vi "Multi_Read_Single.vi"(6 "Manual Range (1)":dbl=1.0, 7 "Auto Range (T: Enable)":bool=TRUE, 8 "error in":errorcluster, 9 "Absolute Resolution (1E-6)":dbl=1e-06, 10 "Measurement Function (10: Voltage DC)":i32(ring)=10 items=["Continuity", "Current AC", "Current DC", "Diode", "Frequency", "Resistance 4-wire", "Period", "Resistance 2-wire", "Temperature", "Voltage AC", "Voltage DC", "Voltage DC Ratio"], 11 "VISA resource name":refnum<visa-resource-name>) -> (0 "error out":errorcluster, 2 "Measurement":dbl)   [LabVIEW 2015]
doc: "This example shows how to configure a measurement and take a reading."
uses:
  <instrlib>/Agilent 3446X Series/Public/Data/Read (Single Point).vi
  <instrlib>/Agilent 3446X Series/Agilent 3446X Series.lvlib
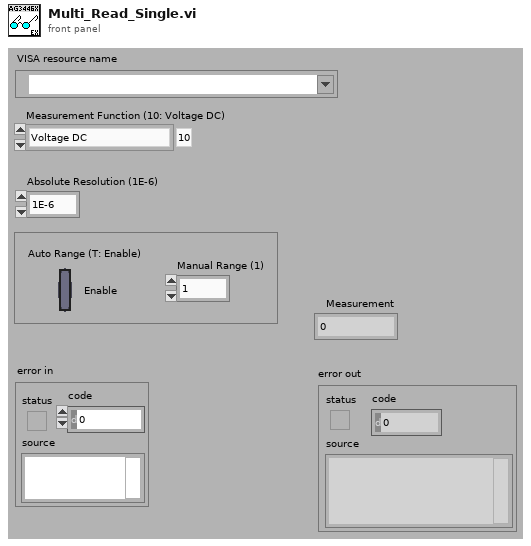
[diagram p1: front panel]
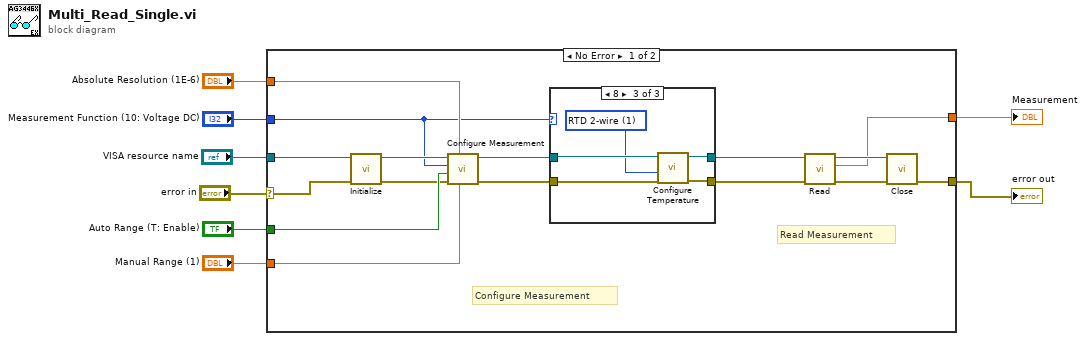
[diagram p0: block diagram]
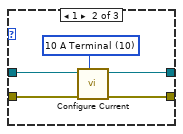
[diagram p3: hidden frame]
diagram:
  n1 = case shown="No Error" "error in" {
    selector: "error in" -> [w16 w37]
    tunnel: [w22 _] -> w8
    tunnel: "Measurement Function (10: Voltage DC)" -> [w9 _]
    tunnel: "Absolute Resolution (1E-6)" -> [w21 _]
    tunnel: "Auto Range (T: Enable)" -> [w20 _]
    tunnel: "Manual Range (1)" -> [w19 _]
    tunnel: "VISA resource name" -> [w18 _]
    tunnel: [w17 w37] -> w2
    frame No Error {
      # "Read Measurement"
      # "Configure Measurement"
      n2 = call <instrlib>:"Initialize.vi"("error in (no error)"=w16, "VISA resource name"=w18) -> ("error out"=w10:errorcluster, "VISA resource name out"=w11:refnum<visa-resource-name>)  [unwired: 3 in, 5 out]
      n3 = call <instrlib>:"Configure Measurement.vi"("Manual Range (1)"=w19, "Absolute Resolution (1E-6)"=w21, "error in (no error)"=w10, "Auto Range (T: Enable)"=w20, "Measurement Function (10: Voltage DC)"=w9, "VISA resource name"=w11) -> ("error out"=w13:errorcluster, "VISA resource name out"=w15:refnum<visa-resource-name>)  [unwired: 4 out]
      n4 = case shown="8" w9 {
        tunnel: w15 -> [w26 w30 w36]
        tunnel: [w26 w29 w32] -> w14
        tunnel: w13 -> [w25 w28 w34]
        tunnel: [w25 w27 w33] -> w12
        frame 0, Default {
        }
        frame 1 {
          w31 = 10 items=["3 A Terminal"=3, "10 A Terminal"=10] ("Terminal Type (3: 3 A Terminal)")
          n5 = call <instrlib>:"Configure Current.vi"("Terminal Type (3: 3 A Terminal)"=w31, "error in (no error)"=w28, "VISA resource name"=w30) -> ("error out"=w27:errorcluster, "VISA resource name out"=w29:refnum<visa-resource-name>)  [unwired: 7 in]
        }
        frame 8 {
          w35 = 1 items=["RTD 4-wire", "RTD 2-wire", "Thermistor 4-wire", "Thermistor 2-wire", "Thermocouple"] ("Probe Type (0: RTD 4-wire)")
          n6 = call <instrlib>:"Configure Temperature.vi"("error in (no error)"=w34, "Probe Type (0: RTD 4-wire)"=w35, "VISA resource name"=w36) -> ("error out"=w33:errorcluster, "VISA resource name out"=w32:refnum<visa-resource-name>)  [unwired: 7 in]
        }
      }
      n7 = call-poly <instrlib>:"Read.vi"("error in (no error)"=w12, "VISA resource name"=w14) -> ("error out"=w24:errorcluster, "Measurement"=w22:dbl, "VISA resource name out"=w23:refnum<visa-resource-name>)  [unwired: 7 out]
      n8 = call <instrlib>:"Close.vi"("error in (no error)"=w24, "VISA resource name"=w23) -> ("error out"=w17:errorcluster)  [unwired: 9 out]
    }
    frame Error {
    }
  }
  "Measurement" <- w8
  "error out" <- w2
